vi "Open Device Info.vi"(8 "error in":errorcluster, 11 "File Path":path) -> (0 "error out":errorcluster, 3 "array of devices":T1)   [LabVIEW 2016]
uses:
  Array Device Info.ctl
  Device Info.ctl
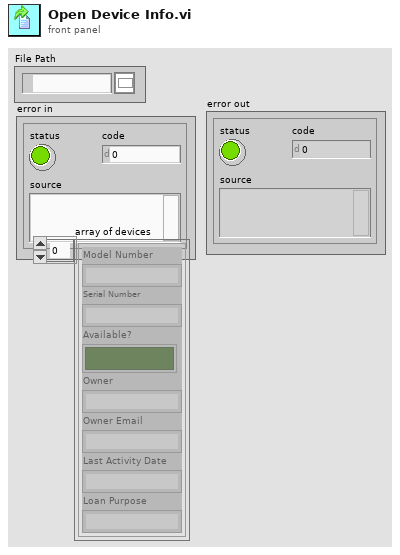
[diagram p1: front panel]
types:
  T1 = typedef "Array Device Info.ctl" = T2[]
  T2 = typedef "Device Info.ctl" = cluster{"Model Number":string, "Serial Number":string, "Available?":bool, "Owner":string, "Owner Email":string, "Last Activity Date":string, "Loan Purpose":string}
  T3 = enum16{"open", "replace", "create", "open or create", "replace or create", "replace or create with confirmation"}
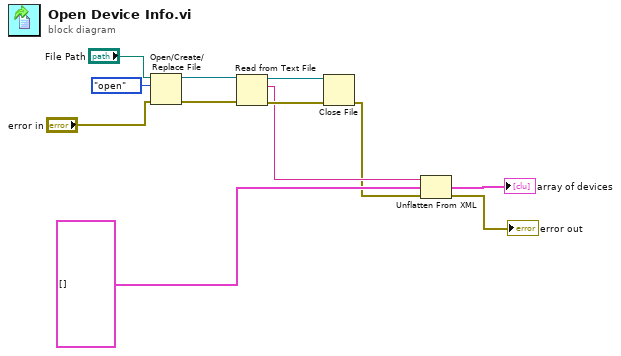
[diagram p0: block diagram]
diagram:
  n1 = Open/Create/Replace File(file path (use dialog)="File Path", error in="error in", operation (0:open)=T3."open") -> (refnum out=w12:refnum<file>, error out=w10:errorcluster)  [unwired: 3 in, 1 out]
  n2 = Read from Text File(file (use dialog)=w12, error in=w10) -> (refnum out=w11:refnum<file>, text=w8:string, error out=w9:errorcluster)  [unwired: 2 in, 1 out]
  n3 = Close File(refnum=w11, error in=w9) -> (error out=w4:errorcluster)  [unwired: 1 out]
  n4 = Unflatten From XML(xml string=w8, type=T1 [] ("Array of Device Info"), error in (no error)=w4) -> (value=→"array of devices":T1, error out=→"error out":errorcluster)
